vi "GUNSC_LibAddAmp.vi"(1 "correctedxstart":i32, 2 "correctedystart":i32, 5 "Amplifier":T1={"number"=0, "type"=0, "rotated"=0, "fliped"=0, "FPAcoord"={"xstart"=1, "ystart"=1}, "Physical_size"={"columns"=0, "rows"=0}, "predata"={"columns"=0, "rows"=0}, "postdata"={"columns"=0, "rows"=0}, "Req ROIs"=[], "Corr ROI"=[], "Detnumber"=0, "ampID"="", "discard"=0} {"fliped" items=["none", "horizontal", "vertical"]; "type" items=["LL", "LR", "UL", "UR"]}, 7 "extension":i32, 11 "error in (no error)":errorcluster, 12 "xdata":i32, 13 "ydata":i32) -> (6 "return value":i32, 15 "error out":errorcluster)   [LabVIEW 2016]
uses:
  GEOM/private/vis/GEOM_Amplifier.ctl
  GEOM/private/vis/GEOM_AmpType.ctl
  GEOM/private/vis/GEOM_ROI.ctl
  GEOM/private/vis/GEOM_Coords.ctl
  public/c/lib/libunsc.so
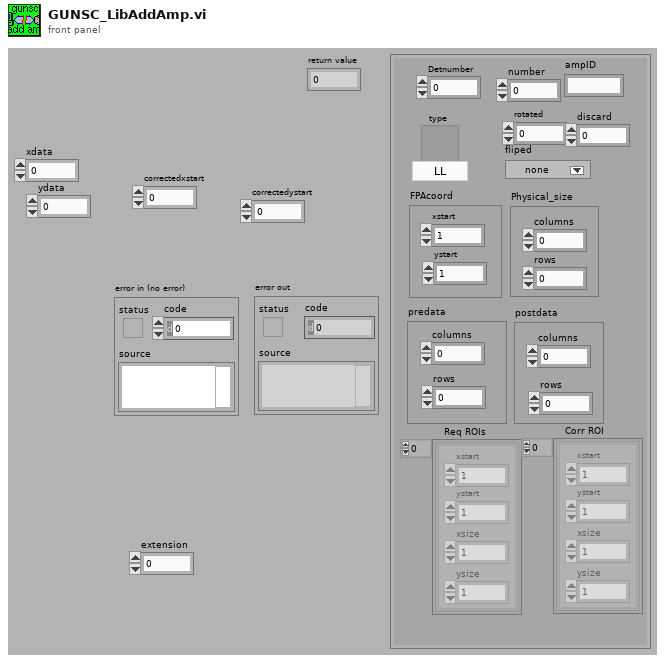
[diagram p1: front panel]
types:
  T1 = typedef "GEOM_Amplifier.ctl" = cluster{"number":i32, "type":T2, "rotated":i16, "fliped":u16, "FPAcoord":cluster{"xstart":i32, "ystart":i32}, "Physical_size":cluster{"columns":i32, "rows":i32}, "predata":cluster{"columns":i32, "rows":i32}, "postdata":cluster{"columns":i32, "rows":i32}, "Req ROIs":T3, "Corr ROI":T3, "Detnumber":i32, "ampID":string, "discard":i32}
  T2 = typedef "GEOM_AmpType.ctl" = u16
  T3 = typedef "GEOM_ROI.ctl" = T4[]
  T4 = typedef "GEOM_Coords.ctl" = cluster{"xstart":u32, "ystart":u32, "xsize":u32, "ysize":u32}
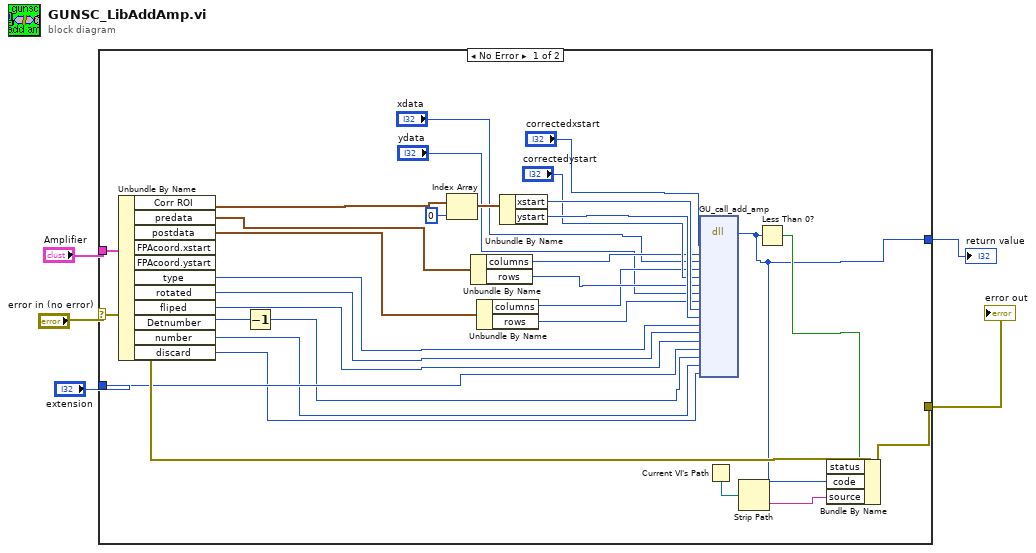
[diagram p0: block diagram]
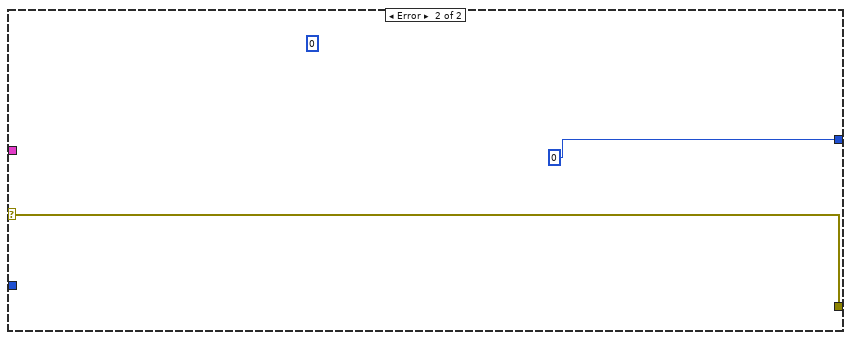
[diagram p2: hidden frame]
diagram:
  n1 = case shown="No Error" "error in (no error)" {
    selector: "error in (no error)" -> [w35 w37]
    tunnel: [w26 0] -> w5
    tunnel: [w32 w37] -> w3
    tunnel: "Amplifier" -> [w31 _]
    tunnel: "extension" -> [w25 _]
    frame No Error {
      n2 = Unbundle By Name(w31) -> ("Corr ROI"=w18:T3, "predata"=w15:cluster{"columns":i32, "rows":i32}, "postdata"=w12:cluster{"columns":i32, "rows":i32}, "type"=w29:T2, "rotated"=w28:i16, "fliped"=w27:u16, "Detnumber"=w9:i32, "number"=w8:i32, "discard"=w6:i32)  [unwired: 2 out]
      n3 = Decrement(x=w9) -> (x-1=w7:i32)
      n4 = Index Array(array=w18, index=0) -> (element=w23:T4)
      n5 = Unbundle By Name(w15) -> ("columns"=w17:i32, "rows"=w16:i32)
      n6 = Unbundle By Name(w12) -> ("columns"=w14:i32, "rows"=w13:i32)
      n7 = Unbundle By Name(w23) -> ("xstart"=w22:u32, "ystart"=w21:u32)
      n8 = dll-call lib="home/simager/panview/PAN/Modules/GUNSC/public/c/lib/libunsc.so" fn="GU_call_add_amp"("xstart"="correctedxstart", "precols"=w17, "datacols"="xdata", "postcols"=w14, "ystart"="correctedystart", "prerows"=w16, "datarows"="ydata", "postrows"=w13, "xdetstart"=w22, "ydetstart"=w21, "type"=w29, "rotate"=w28, "flip"=w27, "extension"=w25, "detno"=w7, "ampno"=w8, "discard"=w6) -> ("return type"=w26:i32)  [unwired: 19 in, 3 out]
      n9 = Current VI's Path() -> (path=w34:path)
      n10 = Strip Path(path=w34) -> (name=w33:string)  [unwired: 1 out]
      n11 = Less Than 0?(x=w26) -> (x < 0?=w30:bool)
      n12 = Bundle By Name(cluster=w35, "status"=w30, "code"=w26, "source"=w33) -> (w32:errorcluster)
    }
    frame Error {
      (unwired) 0
    }
  }
  "return value" <- w5
  "error out" <- w3
